vi "EDEG.vi"(11 "State":i32) -> (3 "EDEG":dbl)   [LabVIEW 2020]
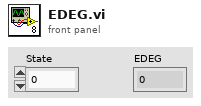
[diagram p1: front panel]
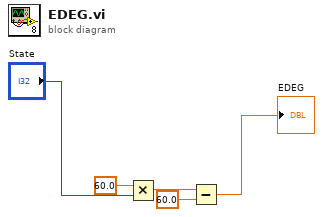
[diagram p0: block diagram]
diagram:
  n1 = Multiply(x=60.0, y="State") -> (x*y=w3:dbl)
  n2 = Subtract(x=w3, y=60.0) -> (x-y=→"EDEG":dbl)
